vi "String PN.vi"(8 "error in (no error)":errorcluster, 10 "Strings []":string[](array[string]), 11 "reference":refnum<vi>) -> (0 "error out":errorcluster, 3 "reference out":refnum<vi>)   [LabVIEW 2022 SP3]
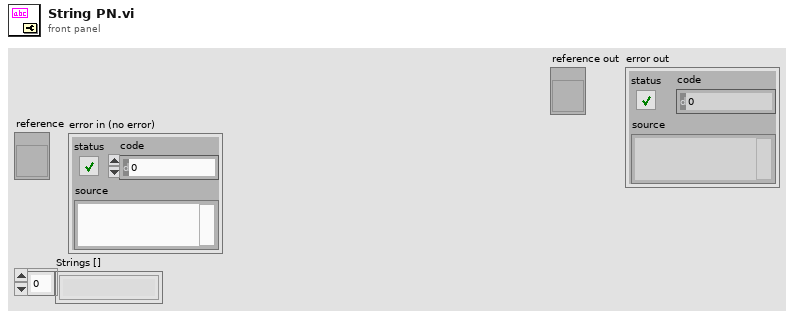
[diagram p1: front panel]
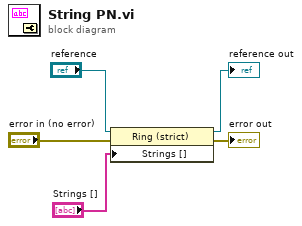
[diagram p0: block diagram]
diagram:
  n1 = property class="Ring (strict)"(reference="reference", error in="error in (no error)", "Strings []"="Strings []") -> (reference out=→"reference out":refnum<vi>, error out=→"error out":errorcluster)
